vi "LP Simplex Method Inner Part.vi"(0 "M":dbl[][](array[numeric]) format="%.2f", 1 "B modified":dbl[](array[numeric]) format="%.2f", 2 "first length M":i32, 3 "second length M":i32, 4 "C":dbl[](array[numeric]) format="%.2f") -> (5 "table*":dbl[][](array[numeric]) format="%.2f", 6 "m*":u32[](array[numeric]), 7 "length of array":i32, 8 "error":i32)   [LabVIEW 2017, in "NI_Gmath.lvlib"]
uses:
  <vilib>/gmath/NI_Gmath.lvlib
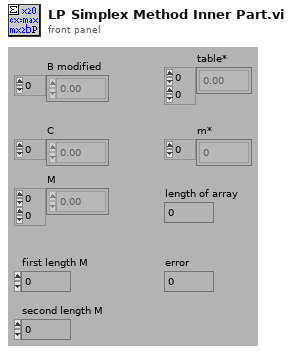
[diagram p1: front panel]
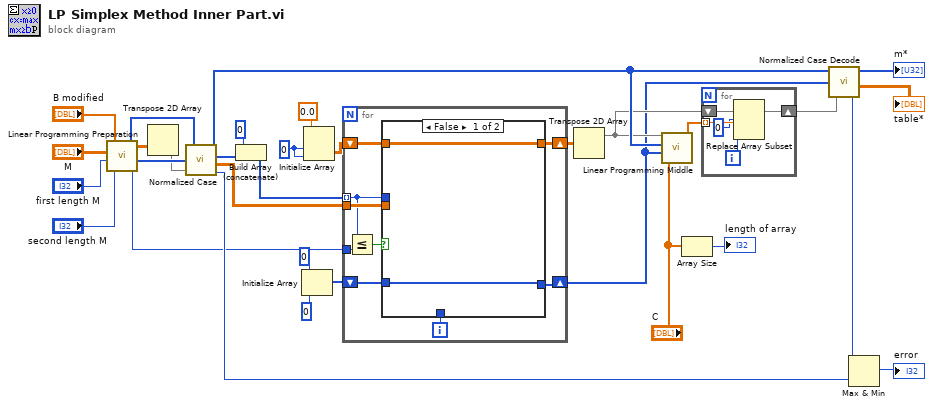
[diagram p0: block diagram]
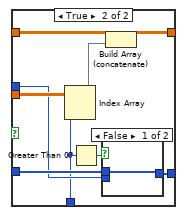
[diagram p2: hidden frame]
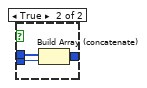
[diagram p3: hidden frame]
diagram:
  w21 = 0
  n1 = call <vilib>:"Linear Programming Preparation.vi"("dim2(M)"="second length M", "dim1 (M)"="first length M", "M"="M", "B"="B modified") -> ("dim1+dim2"=w13:i32, "n-m"=w26:u32[], "m"=w1:u32[], "Table"=w25:dbl[][])
  n2 = Transpose 2D Array(2D array=w25) -> (transposed array=w24:dbl[][])
  n3 = call <vilib>:"Normalized Case.vi"("m"=w1, "n-m"=w26, "table"=w24) -> ("m*"=w32:u32[], "n-m*"=w16:u32[], "table*"=w17:dbl[][], "error"=w29:i32)
  n4 = Build Array (concatenate)(0, w16) -> (w14:u32[])
  n5 = Initialize Array(0, 0) -> (w10:i32[])
  n6 = Initialize Array(0.0, w21, w21) -> (w20:dbl[][])
  n7 = for {
    tunnel: w14 -> [w33] mode=indexing
    tunnel: w13 -> [w41]
    tunnel: w17 -> [w40]
    shift-right: [w38] -> w18
    shift-left: w20 -> [w39]
    shift-right: [w34] -> w6
    shift-left: w10 -> [w35]
    i -> [w36]
    n8 = Less Or Equal?(x=w33, y=w41) -> (x <= y?=w37:bool)
    n9 = case shown="False" w37 {
      tunnel: w40 -> [_ w52]
      tunnel: w36 -> [_ w45]
      tunnel: w39 -> [w43 w51]
      tunnel: [w43 w50] -> w38
      tunnel: w35 -> [w42 w48]
      tunnel: [w42 w47] -> w34
      tunnel: w33 -> [_ w46]
      frame False {
      }
      frame True {
        n10 = Index Array(array=w52, index (col)=w45) -> (element=w49:dbl[])  [unwired: 1 in]
        n11 = Greater Than 0?(x=w45) -> (x > 0?=w44:bool)
        n12 = case shown="False" w44 {
          tunnel: w46 -> [_ w56]
          tunnel: [w53 w55] -> w47
          tunnel: w48 -> [w53 w54]
          frame False {
          }
          frame True {
            n13 = Build Array (concatenate)(w54, w56) -> (w55:u32[])
          }
        }
        n14 = Build Array (concatenate)(w51, w49) -> (w50:dbl[][])
      }
    }
  }
  n15 = Transpose 2D Array(2D array=w18) -> (transposed array=w9:dbl[][])
  n16 = call <vilib>:"Linear Programming Middle.vi"("C"="C", "n-m*"=w6, "m*"=w32, "Table"=w9) -> ("Vector"=w7:dbl[])
  n17 = Array Size(array="C") -> (size(s)=→"length of array":i32)
  n18 = for {
    shift-right: [w57] -> w8
    shift-left: w9 -> [w61]
    tunnel: w7 -> [w60] mode=indexing
    i -> [w59]
    n19 = Replace Array Subset(array=w61, new element=w60, index (row)=0, index (col)=w59) -> (w57:dbl[][])
  }
  n20 = call <vilib>:"Normalized Case Decode.vi"("m"=w32, "n-m"=w6, "table"=w8) -> ("m*"=→"m*":u32[], "table*"=→"table*":dbl[][], "error"=w30:i32)  [unwired: 1 out]
  n21 = Max & Min(x=w30, y=w29) -> (min(x,y)=→"error":i32)  [unwired: 1 out]
